vi "SUMMER SUNDAY FINAL.vi"() -> ()   [LabVIEW 2009]
uses:
  <vilib>/ULx/Create Channel.llb/ULx Create Channel (AI-Voltage-Basic).vi
  <vilib>/ULx/Create Channel.llb/ULx Create Channel (DO-Digital Output).vi
  <vilib>/ULx/Create Channel.llb/ULx Create Channel (DI-Digital Input).vi
  <vilib>/ULx/Write.llb/ULx Write (Digital Bool 1Line 1Point).vi
  <vilib>/ULx/Read.llb/ULx Read (Analog DBL 1Chan 1Samp).vi
  <vilib>/ULx/Read.llb/ULx Read (Digital 1D U8 NChan 1Samp).vi
panel:
  out "max value":u8
  out "POWER":bool
  out "data":dbl format="%_6g"
  out "ENERGY LEVEL":dbl(knob) scale=0.0..15.0
  out "Beam Pot":dbl format="%_6g"
  out "READY 2":bool
  out "DUMP":bool
  out "POWER":bool
  out "?":bool
  out "?":bool
  out "?":bool
  out "?":bool
  out "?":bool
  out "?":bool
  out "?":bool
  out "?":bool
  out "?":bool
  out "?":bool
  out "OPEN":bool
  out "CLOSED":bool
  out "READY":bool
  out "FAULT":bool
  out "MAGNET FORCE":dbl(slide) scale=0.0..10.0
  out "READY":bool
  out "TEMPERATURE":dbl(slide) scale=0.0..100.0
  in  "stop":bool
  out "?":bool
  out "?":bool
  out "?":bool
  out "?":bool
  out "FAULT":bool
  out "POWER":bool
  out "FLOW IN GPM":dbl(knob) scale=0.0..15.0
  # "USERS LAB AREA"
  # "BEAM STATUS"
  # "ROOM"
  # "XRAY"
  # "PUMP STATION"
  # "MAGNET STATUS"
  # "ORBIT"
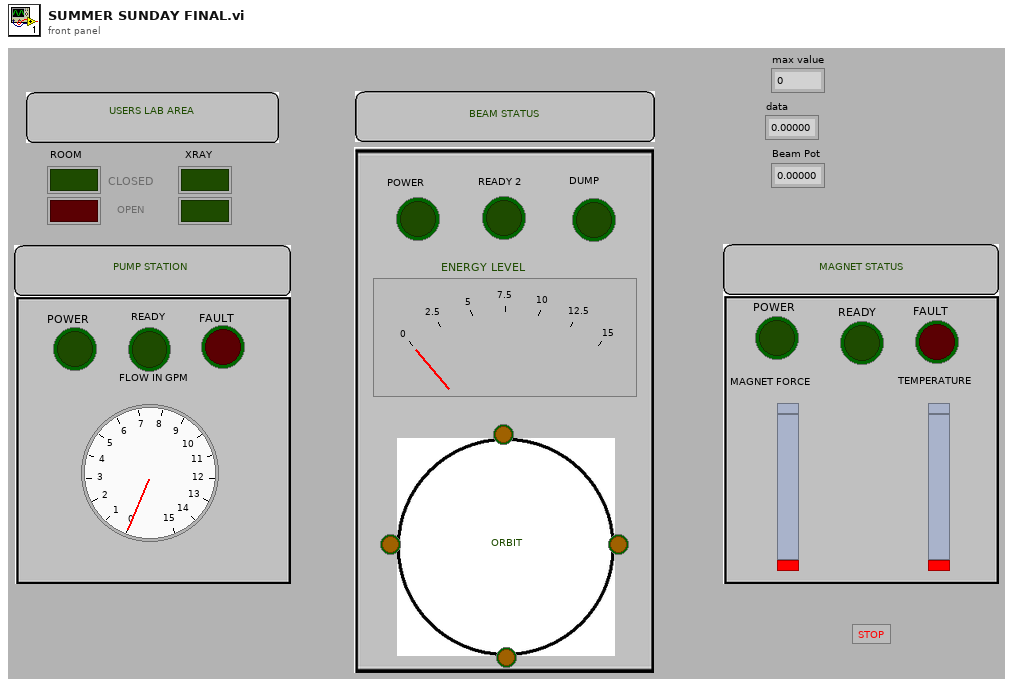
[diagram p1: front panel]
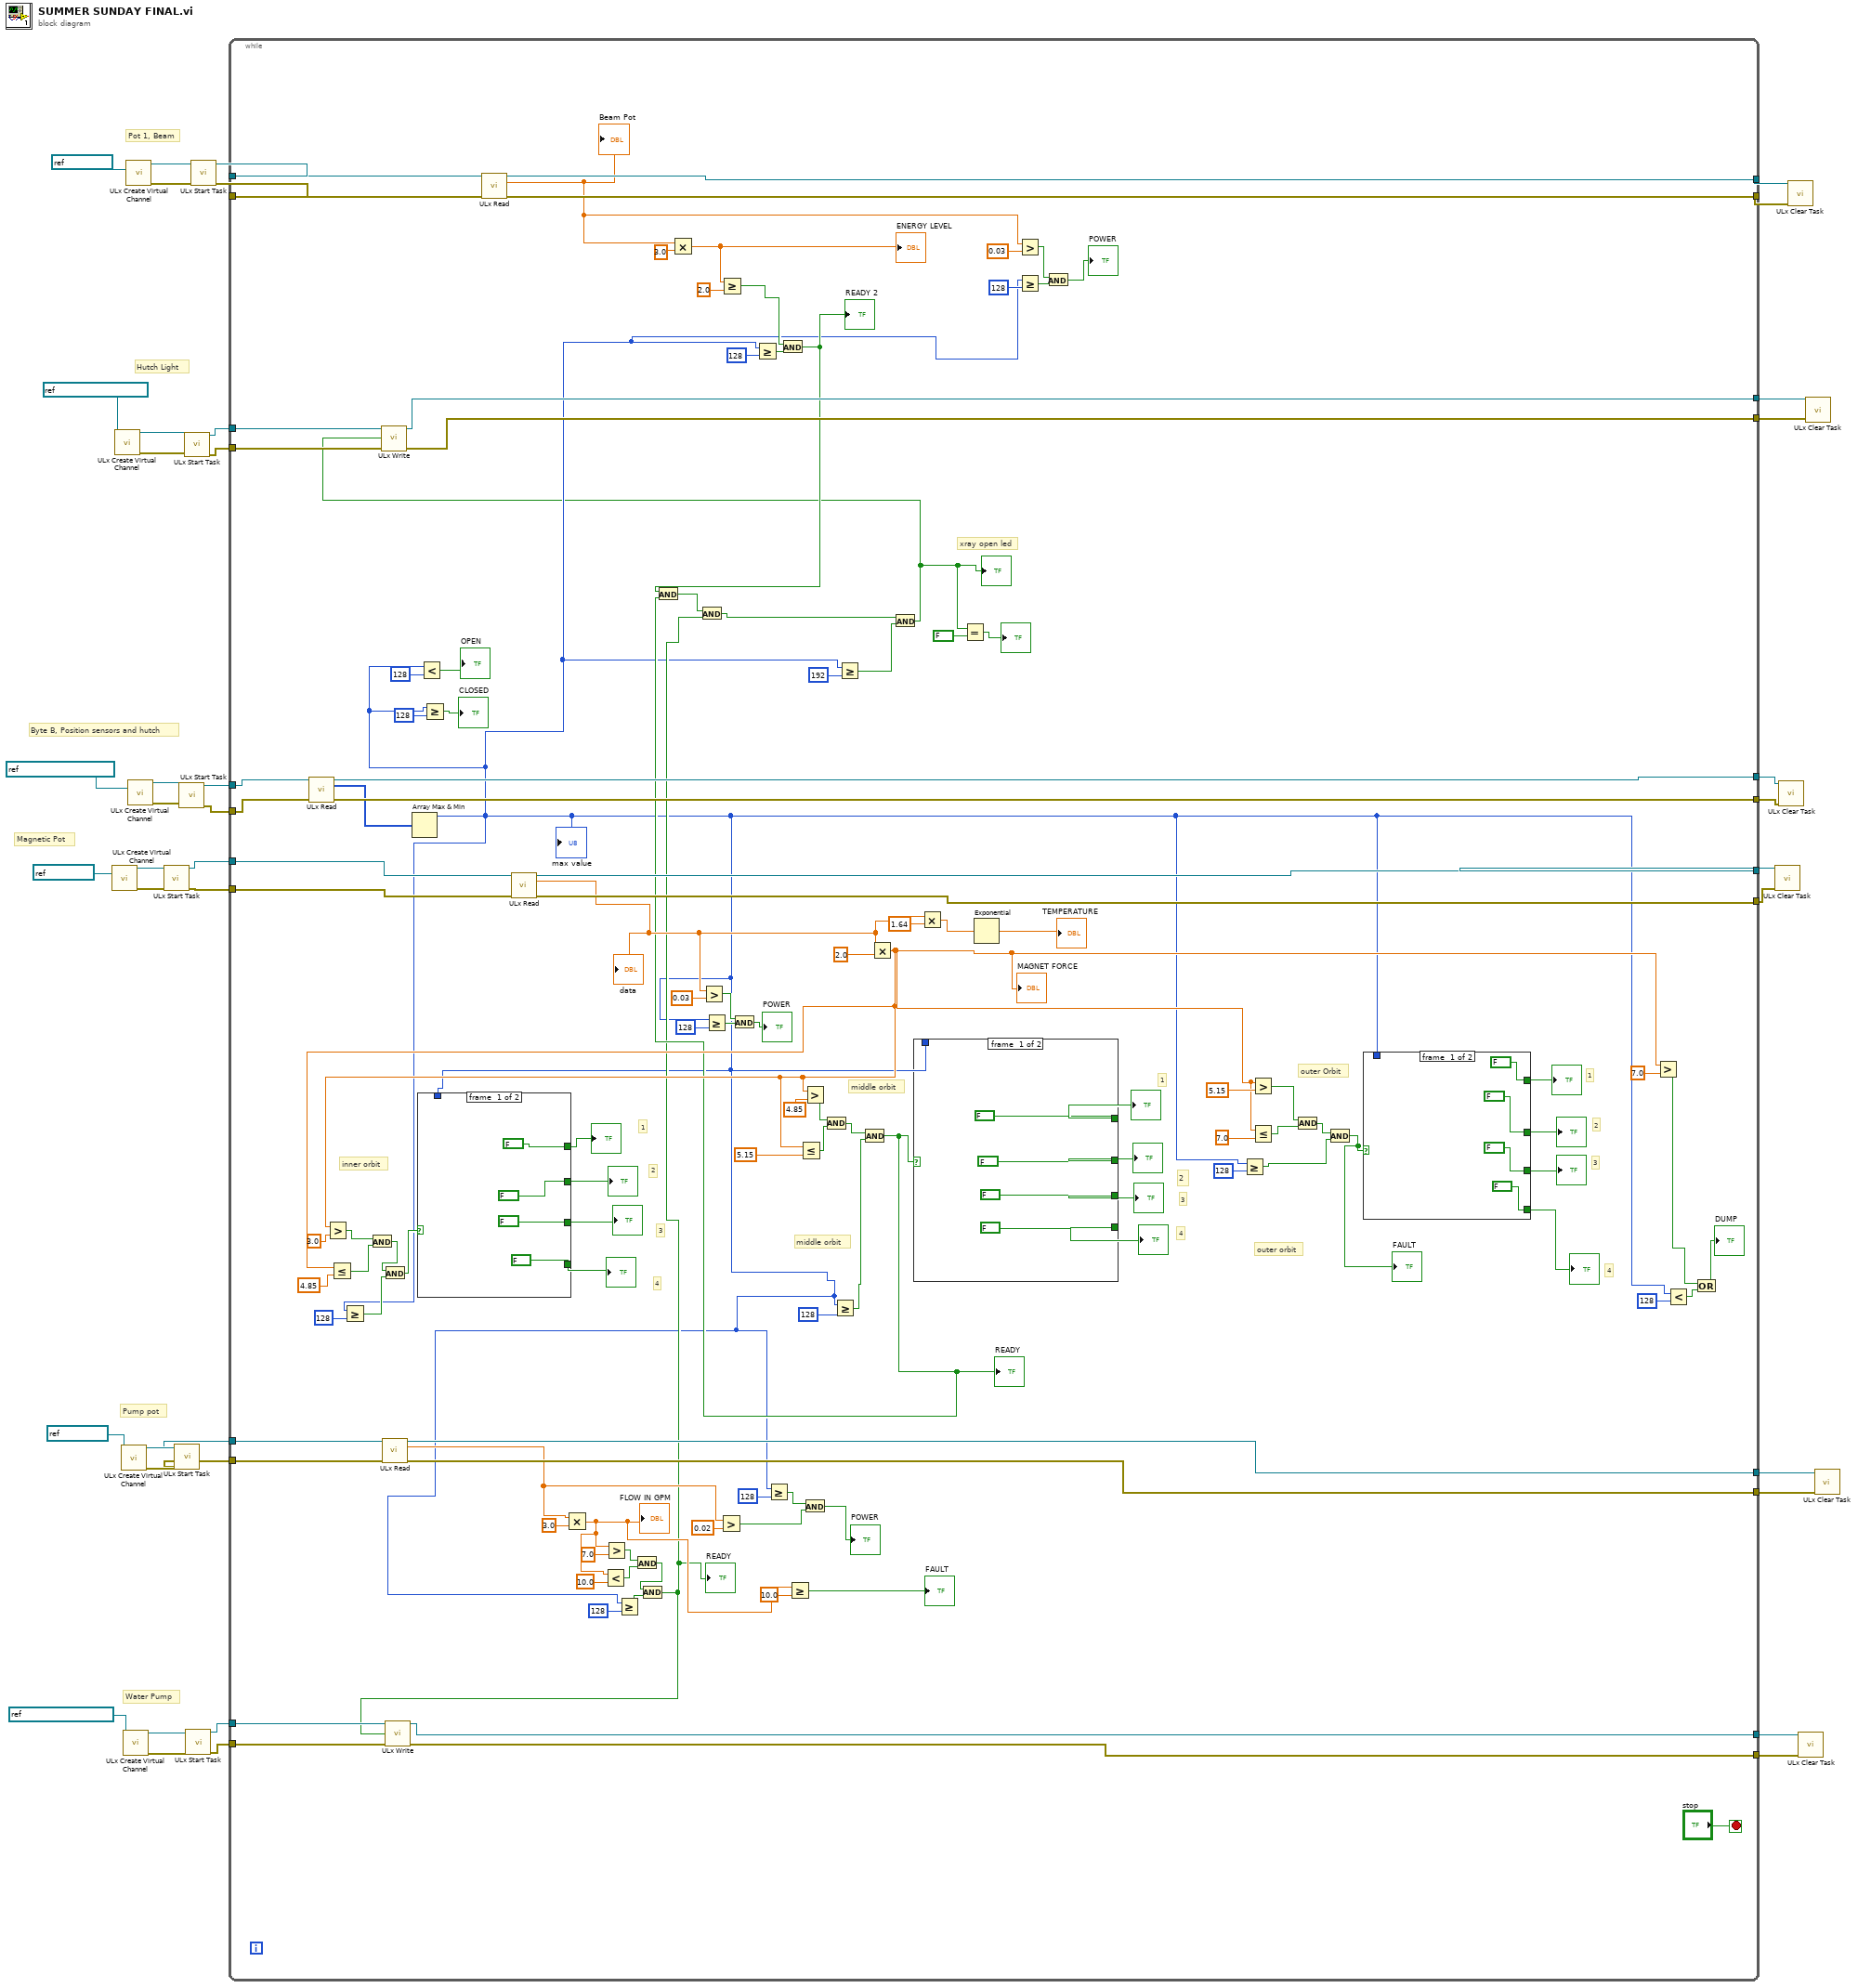
[diagram p0: block diagram]
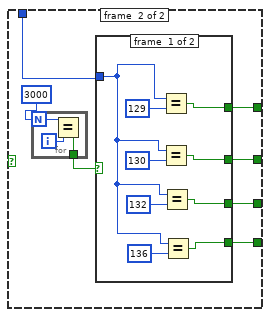
[diagram p2: hidden frame]
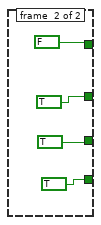
[diagram p3: hidden frame]
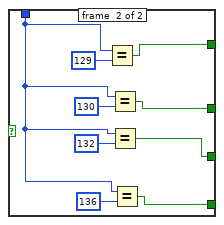
[diagram p4: hidden frame]
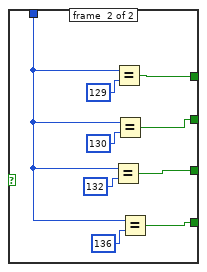
[diagram p5: hidden frame]
diagram:
  # "Water Pump"
  # "Pump pot"
  # "Hutch Light"
  # "Byte B, Position sensors and hutch"
  # "Magnetic Pot"
  # "Pot 1, Beam"
  n1 = call-poly <vilib>:"ULx Create Virtual Channel.vi"("physical channels"=refnum<k21> "Dev0/Ai1") -> ("task out"=w36:refnum<k24>, "error out"=w35:errorcluster)  [unwired: 13 in]
  n2 = call-poly <vilib>:"ULx Create Virtual Channel.vi"("lines"=refnum<k21> "Dev0/1stPortA/Do0") -> ("task out"=w21:refnum<k24>, "error out"=w20:errorcluster)  [unwired: 13 in]
  n3 = call-poly <vilib>:"ULx Create Virtual Channel.vi"("physical channels"=refnum<k21> "Dev0/Ai2") -> ("task out"=w28:refnum<k24>, "error out"=w27:errorcluster)  [unwired: 13 in]
  n4 = call-poly <vilib>:"ULx Create Virtual Channel.vi"("lines"=refnum<k21> "Dev0/1stPortA/Do1") -> ("task out"=w7:refnum<k24>, "error out"=w6:errorcluster)  [unwired: 13 in]
  n5 = call-poly <vilib>:"ULx Create Virtual Channel.vi"("physical channels"=refnum<k21> "Dev0/Ai0") -> ("task out"=w42:refnum<k24>, "error out"=w41:errorcluster)  [unwired: 13 in]
  n6 = call-poly <vilib>:"ULx Create Virtual Channel.vi"("lines"=refnum<k21> "Dev0/1stPortB/Di0:7") -> ("task out"=w14:refnum<k24>, "error out"=w13:errorcluster)  [unwired: 13 in]
  n7 = call <vilib>:"ULx Start Task.vi"("task in"=w36, "error in"=w35) -> ("task out"=w34:refnum<k24>, "error out"=w33:errorcluster)  [unwired: 12 in]
  n8 = call <vilib>:"ULx Start Task.vi"("task in"=w28, "error in"=w27) -> ("task out"=w26:refnum<k24>, "error out"=w25:errorcluster)  [unwired: 12 in]
  n9 = call <vilib>:"ULx Start Task.vi"("task in"=w14, "error in"=w13) -> ("task out"=w12:refnum<k24>, "error out"=w11:errorcluster)  [unwired: 12 in]
  n10 = call <vilib>:"ULx Start Task.vi"("task in"=w21, "error in"=w20) -> ("task out"=w18:refnum<k24>, "error out"=w17:errorcluster)  [unwired: 12 in]
  n11 = call <vilib>:"ULx Start Task.vi"("task in"=w7, "error in"=w6) -> ("task out"=w5:refnum<k24>, "error out"=w4:errorcluster)  [unwired: 12 in]
  n12 = call <vilib>:"ULx Start Task.vi"("task in"=w42, "error in"=w41) -> ("task out"=w40:refnum<k24>, "error out"=w39:errorcluster)  [unwired: 12 in]
  n13 = while {
    tunnel: w40 -> [w162]
    tunnel: w39 -> [w161]
    tunnel: [w160] -> w38
    tunnel: [w159] -> w37
    tunnel: w34 -> [w157]
    tunnel: w33 -> [w156]
    tunnel: [w155] -> w32
    tunnel: [w154] -> w31
    tunnel: w26 -> [w116]
    tunnel: w25 -> [w115]
    tunnel: [w114] -> w23
    tunnel: [w113] -> w22
    tunnel: w18 -> [w91]
    tunnel: w17 -> [w90]
    tunnel: [w89] -> w16
    tunnel: [w88] -> w15
    tunnel: w12 -> [w87]
    tunnel: w11 -> [w86]
    tunnel: [w85] -> w9
    tunnel: [w84] -> w8
    tunnel: w5 -> [w59]
    tunnel: w4 -> [w58]
    tunnel: [w57] -> w3
    tunnel: [w56] -> w2
    stop <- "stop" stop-if-true
    # "xray open led"
    # "outer Orbit"
    # "middle orbit"
    # "4"
    # "3"
    # "2"
    # "1"
    # "1"
    # "2"
    # "3"
    # "4"
    # "4"
    # "3"
    # "2"
    # "1"
    # "outer orbit"
    # "inner orbit"
    # "middle orbit"
    n14 = call-poly <vilib>:"ULx Read.vi"("task in"=w87, "error in"=w86) -> ("task out"=w85:refnum<k24>, "data"=w83:u8[], "error out"=w84:errorcluster)  [unwired: 11 in]
    n15 = call-poly <vilib>:"ULx Read.vi"("task in"=w116, "error in"=w115) -> ("task out"=w114:refnum<k24>, "data"=w109:dbl, "error out"=w113:errorcluster)  [unwired: 11 in]
    n16 = Array Max & Min(array=w83) -> (max value=w47:u8)  [unwired: 3 out]
    "max value" <- w47
    n17 = Greater Or Equal?(x=w47, y=i16 128) -> (x >= y?=w141:bool)
    n18 = Less?(x=w47, y=u8 128) -> (x < y?=→"OPEN":bool)
    n19 = Greater Or Equal?(x=w47, y=u8 128) -> (x >= y?=→"CLOSED":bool)
    n20 = call-poly <vilib>:"ULx Read.vi"("task in"=w162, "error in"=w161) -> ("task out"=w160:refnum<k24>, "data"=w49:dbl, "error out"=w159:errorcluster)  [unwired: 11 in]
    "Beam Pot" <- w49
    n21 = call-poly <vilib>:"ULx Read.vi"("task in"=w157, "error in"=w156) -> ("task out"=w155:refnum<k24>, "data"=w95:dbl, "error out"=w154:errorcluster)  [unwired: 11 in]
    "data" <- w95
    n22 = Multiply(x=w109, y=3.0) -> (x*y=w101:dbl)
    "FLOW IN GPM" <- w101
    n23 = Less?(x=w101, y=10.0) -> (x < y?=w99:bool)
    n24 = Greater?(x=w101, y=7.0) -> (0:w100:bool)
    n25 = Greater Or Equal?(x=w47, y=u8 128) -> (x >= y?=w73:bool)
    n26 = And(x=w100, y=w99) -> (x .and. y?=w71:bool)
    n27 = And(x=w71, y=w73) -> (x .and. y?=w51:bool)
    "READY" <- w51
    n28 = call-poly <vilib>:"ULx Write.vi"("task in"=w59, "data"=w51, "error in"=w58) -> ("task out"=w57:refnum<k24>, "error out"=w56:errorcluster)  [unwired: 10 in, 1 out]
    n29 = Multiply(x=w49, y=3.0) -> (x*y=w106:dbl)
    "ENERGY LEVEL" <- w106
    n30 = Greater?(x=w95, y=0.03) -> (0:w76:bool)
    n31 = Greater Or Equal?(x=w47, y=u8 128) -> (x >= y?=w75:bool)
    n32 = Greater?(x=w109, y=0.02) -> (0:w68:bool)
    n33 = Greater Or Equal?(x=w106, y=2.0) -> (x >= y?=w48:bool)
    n34 = And(x=w76, y=w75) -> (x .and. y?=→"POWER":bool)
    n35 = Greater Or Equal?(x=w47, y=u8 128) -> (x >= y?=w65:bool)
    n36 = Greater Or Equal?(x=w47, y=u8 128) -> (x >= y?=w69:bool)
    n37 = And(x=w48, y=w65) -> (x .and. y?=w63:bool)
    "READY 2" <- w63
    n38 = Greater Or Equal?(x=w101, y=10.0) -> (x >= y?=→"FAULT":bool)
    n39 = And(x=w69, y=w68) -> (x .and. y?=→"POWER":bool)
    n40 = Greater Or Equal?(x=w47, y=i16 128) -> (x >= y?=w82:bool)
    n41 = Greater Or Equal?(x=w47, y=u8 192) -> (x >= y?=w77:bool)
    n42 = Multiply(x=w95, y=2.0) -> (x*y=w134:dbl)
    "MAGNET FORCE" <- w134
    n43 = Greater?(x=w134, y=3.0) -> (0:w150:bool)
    n44 = Less Or Equal?(x=w134, y=4.85) -> (x <= y?=w151:bool)
    n45 = And(x=w150, y=w151) -> (x .and. y?=w143:bool)
    n46 = And(x=w143, y=w141) -> (x .and. y?=w142:bool)
    n47 = case shown="True" w142 {
      tunnel: [FALSE w211] -> w119
      tunnel: [FALSE w210] -> w120
      tunnel: [FALSE w209] -> w117
      tunnel: [FALSE w208] -> w118
      tunnel: w47 -> [_ w216]
      frame #0 {
      }
      frame #1 {
        n48 = Equal?(x=w216, y=i16 132) -> (x = y?=w209:bool)
        n49 = Equal?(x=w216, y=i16 129) -> (x = y?=w211:bool)
        n50 = Equal?(x=w216, y=i16 130) -> (x = y?=w210:bool)
        n51 = Equal?(x=w216, y=i16 136) -> (x = y?=w208:bool)
      }
    }
    "?" <- w120
    "?" <- w117
    "?" <- w118
    "?" <- w119
    n52 = Less Or Equal?(x=w134, y=5.15) -> (x <= y?=w147:bool)
    n53 = Greater?(x=w134, y=4.85) -> (0:w148:bool)
    n54 = And(x=w148, y=w147) -> (x .and. y?=w140:bool)
    n55 = And(x=w140, y=w82) -> (x .and. y?=w80:bool)
    "READY" <- w80
    n56 = And(x=w63, y=w80) -> (x .and. y?=w79:bool)
    n57 = And(x=w79, y=w51) -> (x .and. y?=w78:bool)
    n58 = And(x=w78, y=w77) -> (x .and. y?=w45:bool)
    "?" <- w45
    n59 = call-poly <vilib>:"ULx Write.vi"("task in"=w91, "data"=w45, "error in"=w90) -> ("task out"=w89:refnum<k24>, "error out"=w88:errorcluster)  [unwired: 10 in, 1 out]
    n60 = case shown="True" w80 {
      tunnel: [FALSE w174] -> w129
      tunnel: [FALSE w173] -> w128
      tunnel: [FALSE w172] -> w127
      tunnel: [FALSE w171] -> w126
      tunnel: w47 -> [_ w170]
      frame #0 {
      }
      frame #1 {
        n61 = for {
          N: u32 3000 ("y") -> [w177]
          tunnel: [w175] -> w168
          i -> [w176]
          n62 = Equal?(x=w177, y=w176) -> (x = y?=w175:bool)
        }
        n63 = case shown="False" w168 {
          tunnel: [w181 FALSE] -> w174
          tunnel: [w180 TRUE] -> w173
          tunnel: [w179 TRUE] -> w172
          tunnel: [w178 TRUE] -> w171
          tunnel: w170 -> [w182 _]
          frame #0 {
            n64 = Equal?(x=w182, y=i16 129) -> (x = y?=w181:bool)
            n65 = Equal?(x=w182, y=i16 130) -> (x = y?=w180:bool)
            n66 = Equal?(x=w182, y=i16 132) -> (x = y?=w179:bool)
            n67 = Equal?(x=w182, y=i16 136) -> (x = y?=w178:bool)
          }
          frame #1 {
          }
        }
      }
    }
    "?" <- w129
    "?" <- w128
    "?" <- w127
    "?" <- w126
    n68 = Multiply(x=w95, y=1.64) -> (x*y=w93:dbl)
    n69 = Equal?(x=w45, y=FALSE) -> (x = y?=→"?":bool)
    n70 = Exponential(1:w93) -> (0:→"TEMPERATURE":dbl)
    n71 = Greater?(x=w49, y=0.03) -> (0:w61:bool)
    n72 = Greater Or Equal?(x=w47, y=u8 128) -> (x >= y?=w66:bool)
    n73 = And(x=w61, y=w66) -> (x .and. y?=→"POWER":bool)
    n74 = Greater Or Equal?(x=w47, y=i16 128) -> (x >= y?=w124:bool)
    n75 = Greater?(x=w134, y=5.15) -> (0:w145:bool)
    n76 = Less Or Equal?(x=w134, y=7.0) -> (x <= y?=w144:bool)
    n77 = And(x=w145, y=w144) -> (x .and. y?=w133:bool)
    n78 = And(x=w133, y=w124) -> (x .and. y?=w96:bool)
    "FAULT" <- w96
    n79 = case shown="True" w96 {
      tunnel: [FALSE w195] -> w138
      tunnel: [FALSE w196] -> w137
      tunnel: [FALSE w197] -> w136
      tunnel: [FALSE w198] -> w135
      tunnel: w47 -> [_ w203]
      frame #0 {
      }
      frame #1 {
        n80 = Equal?(x=w203, y=i16 129) -> (x = y?=w198:bool)
        n81 = Equal?(x=w203, y=i16 130) -> (x = y?=w197:bool)
        n82 = Equal?(x=w203, y=i16 132) -> (x = y?=w196:bool)
        n83 = Equal?(x=w203, y=i16 136) -> (x = y?=w195:bool)
      }
    }
    "?" <- w135
    "?" <- w136
    "?" <- w137
    "?" <- w138
    n84 = Greater?(x=w134, y=7.0) -> (0:w97:bool)
    n85 = Less?(x=w47, y=i16 128) -> (x < y?=w121:bool)
    n86 = Or(x=w97, y=w121) -> (x .or. y?=→"DUMP":bool)
  }
  n87 = call <vilib>:"ULx Clear Task.vi"("task in"=w32, "error in"=w31) -> ()  [unwired: 13 in, 1 out]
  n88 = call <vilib>:"ULx Clear Task.vi"("task in"=w9, "error in"=w8) -> ()  [unwired: 13 in, 1 out]
  n89 = call <vilib>:"ULx Clear Task.vi"("task in"=w38, "error in"=w37) -> ()  [unwired: 13 in, 1 out]
  n90 = call <vilib>:"ULx Clear Task.vi"("task in"=w3, "error in"=w2) -> ()  [unwired: 13 in, 1 out]
  n91 = call <vilib>:"ULx Clear Task.vi"("task in"=w16, "error in"=w15) -> ()  [unwired: 13 in, 1 out]
  n92 = call <vilib>:"ULx Clear Task.vi"("task in"=w23, "error in"=w22) -> ()  [unwired: 13 in, 1 out]
